vi "Process Entries.vi"(6 "char limit (2048)":i32=2048, 8 "error in (no error)":errorcluster, 10 "Write to System Log (false)":bool, 11 "Logging in":refnum<class "Logging.lvclass">) -> (0 "error out":errorcluster, 2 "Log text":string, 3 "Logging out":refnum<class "Logging.lvclass">)   [LabVIEW 2020, in "Logging.lvclass"]
uses:
  Logging.lvclass
  Logging.lvclass/Logging.ctl
  <vilib>/Utility/error.llb/DialogType.ctl
  <vilib>/addons/analyzer/_analyzerutils.llb/VIAnUtil Check Type If ErrClust.vi
  <vilib>/Utility/Data Type/NI_Data Type.lvlib
  <vilib>/Utility/SystemLogging/NI_SystemLogging.lvlib
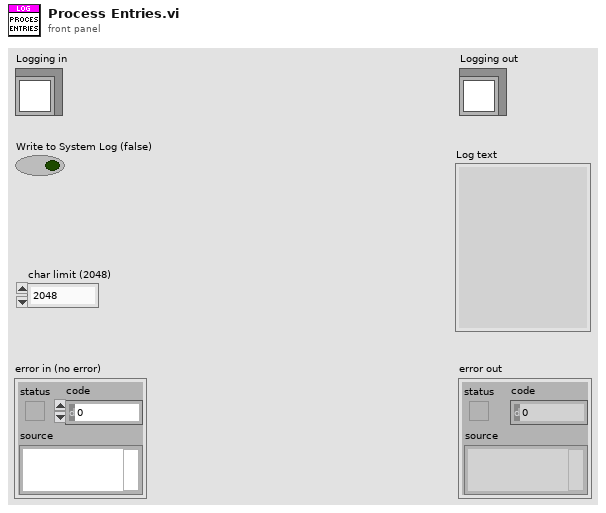
[diagram p1: front panel]
types:
  T1 = typedef "Log entry.ctl" = cluster{"timestamp":timestamp, "data":variant, "origin":string, "severity":i32}
  T2 = typedef "NI_Data Type.lvlib/Data Type.ctl" = enum8{"Invalid Type", "Void", "I8", "I16", "I32", "I64", "U8", "U16", "U32", "U64", "Single Float", "Double Float", "Extended Float", "Single Complex", "Double Complex", "Extended Complex", "Enum U8", "Enum U16", "Enum U32", "Enum U64", "Single Float With Unit", "Double Float With Unit", "Extended Float With Unit", "Single Complex with Unit", "Double Complex with Unit", "Extended Complex with Unit", "Boolean", "String", "Path", "Picture", "Tag", "Array", "Cluster", "Variant", "LV Variant", "Waveform", "Timestamp", "Digital Waveform", "Digital Data", "ExpressData", "Refnum", "External Data", "VI", "Poly VI", "LabVIEW Class Instance", "Fixed Point", "Set Collection", "Map Collection"}
  T3 = typedef "DialogType.ctl" = u16
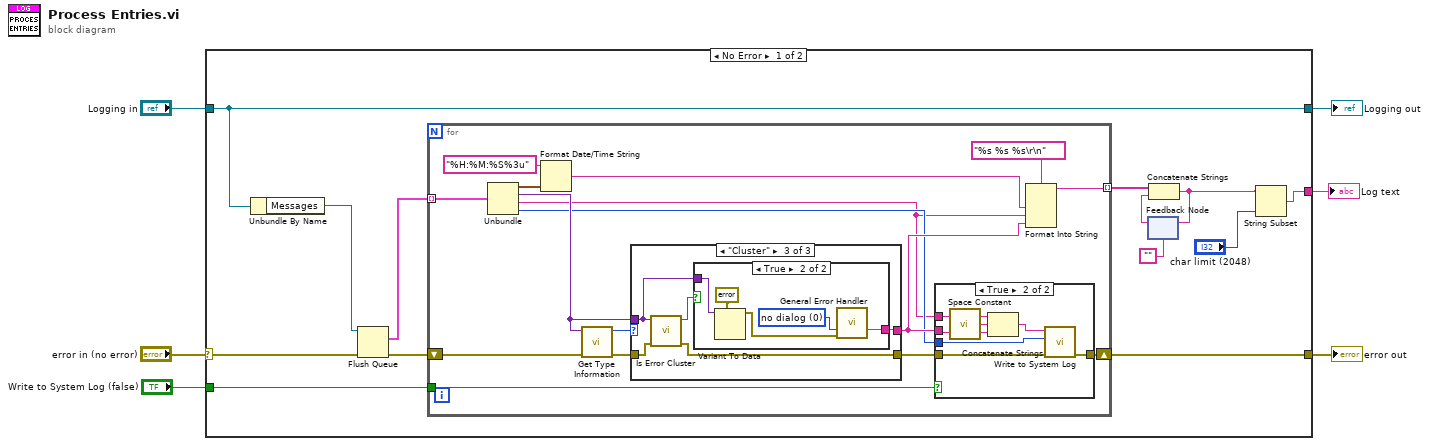
[diagram p0: block diagram]
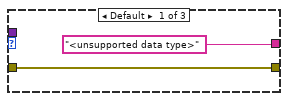
[diagram p3: hidden frame]
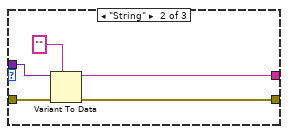
[diagram p4: hidden frame]
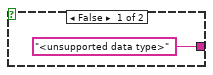
[diagram p5: hidden frame]
diagram:
  n1 = case shown="No Error" "error in (no error)" {
    selector: "error in (no error)" -> [w17 w63]
    tunnel: [w14 w63] -> w5
    tunnel: [w19 w62] -> w3
    tunnel: "Logging in" -> [w19 w62]
    tunnel: [w9 _] -> w2
    tunnel: "Write to System Log (false)" -> [w7 _]
    frame No Error {
      n2 = Unbundle By Name(w19) -> ("Messages"=w18:refnum<queue>)
      n3 = Flush Queue(queue=w18, error in (no error)=w17) -> (remaining elements=w16:T1[], error out=w15:errorcluster)  [unwired: 1 out]
      n4 = for {
        tunnel: w16 -> [w29] mode=indexing
        tunnel: [w27] -> w12 mode=indexing
        tunnel: w7 -> [w24]
        shift-right: [w25] -> w14
        shift-left: w15 -> [w32]
        n5 = Unbundle(w29) -> ("timestamp"=w35:timestamp, "data"=w30:variant, "origin"=w20:string, "severity"=w21:i32)
        n6 = Format Date/Time String(time format string (%c)="%H:%M:%S%3u", seconds (now)=w35) -> (date/time string=w23:string)  [unwired: 1 in]
        n7 = call <vilib>:"Get Type Information.vi"("error in (no error)"=w32, "variant"=w30) -> ("error out"=w31:errorcluster, "type"=w33:T2)  [unwired: 5 in, 3 out]
        n8 = case shown="\"Cluster\"" w33 {
          tunnel: w30 -> [_ w46 w52]
          tunnel: ["<unsupported data type>" w50 w54] -> w22
          tunnel: w31 -> [w45 w48 w55]
          tunnel: [w45 w47 w53] -> w26
          frame Default {
          }
          frame "String" {
            n9 = Variant To Data(error in=w48, type="", Variant=w46) -> (data=w50:string, error out=w47:errorcluster)
          }
          frame "Cluster" {
            n10 = call <vilib>:"Is Error Cluster.vi"("error in (no error)"=w55, "variant"=w52) -> ("error out"=w53:errorcluster, "is error cluster?"=w51:bool)  [unwired: 8 in]
            n11 = case shown="True" w51 {
              tunnel: ["<unsupported data type>" ("format string") w57] -> w54
              tunnel: w52 -> [_ w60]
              frame False {
              }
              frame True {
                w59 = T3 0 items=["no dialog", "OK message", "continue or stop message", "OK message + warnings", "continue/stop + warnings"] ("type of dialog (OK msg:1)")
                n12 = Variant To Data(type=errorcluster {"status"=FALSE, "code"=0, "source"=""} ("error IO"), Variant=w60) -> (data=w58:errorcluster)  [unwired: 1 in, 1 out]
                n13 = call <vilib>:"General Error Handler.vi"("type of dialog (OK msg:1)"=w59, "error in (no error)"=w58) -> ("message"=w57:string)  [unwired: 9 in, 4 out]
              }
            }
          }
        }
        n14 = case shown="True" w24 {
          tunnel: w26 -> [w36 w43]
          tunnel: [w36 w42] -> w25
          tunnel: w22 -> [_ w39]
          tunnel: w21 -> [_ w38]
          tunnel: w20 -> [_ w37]
          frame False {
          }
          frame True {
            n15 = call <vilib>:"Space Constant.vi"() -> ("String"=w41:string)
            n16 = Concatenate Strings(w37, w41, w39) -> (w40:string)
            n17 = call <vilib>:"Write to System Log.vi"("error in (no error)"=w43, "severity"=w38, "message"=w40) -> ("error out"=w42:errorcluster)  [unwired: 8 in]
          }
        }
        n18 = Format Into String(format string="%s %s %s\r\n", w23, w20, w22) -> (resulting string=w27:string)  [unwired: 2 in, 1 out]
      }
      n19 = feedback #1("") -> (w11:string)
      n20 = Concatenate Strings(w12, w11) -> (w10:string)
      n21 = feedback-in #1(w10) -> ()
      n22 = String Subset(string=w10, length (rest)="char limit (2048)") -> (substring=w9:string)  [unwired: 1 in]
    }
    frame Error {
    }
  }
  "error out" <- w5
  "Logging out" <- w3
  "Log text" <- w2
